vi "SetSpeedFine.vi"(8 "error in (no error)":errorcluster, 10 "Speed(0..4095)":u16, 11 "DCMotor in":refnum<class "DCMotor.lvclass">) -> (0 "error out":errorcluster, 3 "DCMotor out":refnum<class "DCMotor.lvclass">)   [LabVIEW 2022 SP3, in "Motorshield.lvlib" / "DCMotor.lvclass"]
uses:
  DCMotor.lvclass
  DCMotor.lvclass/DCMotor.ctl
  Motorshield/Motorshield.lvclass
  C:/Users/Carlos/Desktop/onlab/source/Motorshield/Motorshield/Motorshield.lvclass
  C:/Users/Carlos/Desktop/onlab/source/Motorshield/DCMotor/DCMotor.lvclass
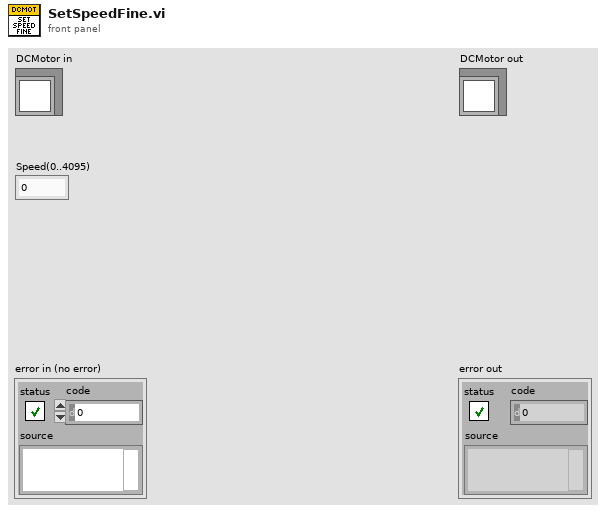
[diagram p1: front panel]
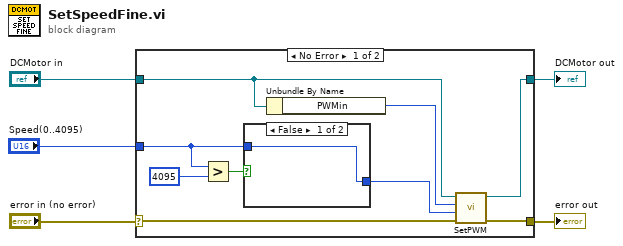
[diagram p0: block diagram]
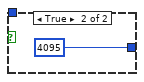
[diagram p2: hidden frame]
diagram:
  n1 = case shown="No Error" "error in (no error)" {
    selector: "error in (no error)" -> [w13 w18]
    tunnel: [w12 w18] -> w4
    tunnel: [w10 w17] -> w2
    tunnel: "DCMotor in" -> [w11 w17]
    tunnel: "Speed(0..4095)" -> [w6 _]
    frame No Error {
      n2 = Greater?(x=w6, y=u16 4095) -> (0:w8:bool)
      n3 = case shown="False" w8 {
        tunnel: [w15 u16 4095 ("y")] -> w7
        tunnel: w6 -> [w15 _]
        frame False {
        }
        frame True {
        }
      }
      n4 = Unbundle By Name(w11) -> ("PWMin"=w14:u8)
      n5 = call "SetPWM.vi"("error in (no error)"=w13, "Value"=w7, "Led num"=w14, "Motorshield in"=w11) -> ("error out"=w12:errorcluster, "Motorshield out"=w10:refnum<class "DCMotor.lvclass">)  [unwired: 6 in]
    }
    frame Error {
    }
  }
  "error out" <- w4
  "DCMotor out" <- w2
